vi "Get Form.vi"(8 "error in (no error)":errorcluster, 11 "Open Form in":refnum<class "Open Form.lvclass">) -> (0 "error out":errorcluster, 2 "Class Path":path, 3 "Open Form out":refnum<class "Open Form.lvclass">)   [LabVIEW 2020, in "Open Form Button.lvlib" / "Open Form.lvclass"]
uses:
  Open Form.lvclass
  Open Form.lvclass/Open Form.ctl
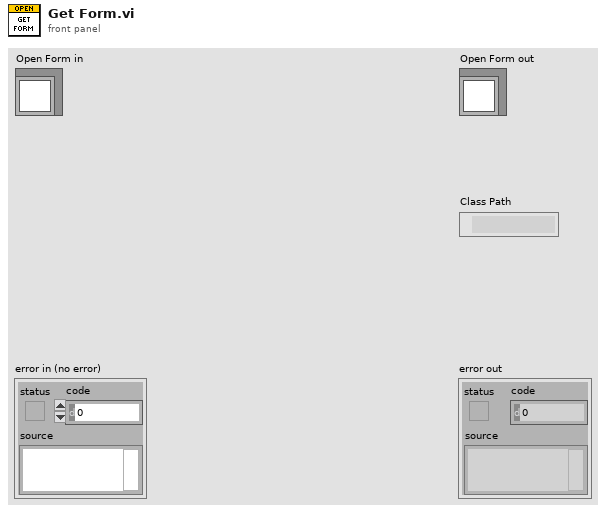
[diagram p1: front panel]
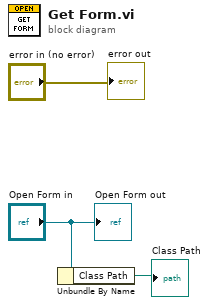
[diagram p0: block diagram]
diagram:
  n1 = Unbundle By Name("Open Form in") -> ("Class Path"=→"Class Path":path)
  "error out" <- "error in (no error)"
  "Open Form out" <- "Open Form in"
